vi "Encode PID Parameters.vi"(8 "ADD Parameters (in)":string, 9 "Scanner Settings In":T2={"Scan1"=1, "Scan2"=1, "Scan3"=1, "Scan4"=1, "Scan5"=1, "Scan6"=1, "Scan7"=1, "Scan8"=1, "Scan9"=1, "Scan10"=1, "Scan11"=1, "Scan12"=1, "Scan13"=1, "Scan14"=1, "Scan15"=1, "Scan16"=1} {"Scan16" scale=0.0..2.0; "Scan15" scale=0.0..2.0; "Scan14" scale=0.0..2.0; "Scan13" scale=0.0..2.0; "Scan12" scale=0.0..2.0; "Scan11" scale=0.0..2.0; "Scan10" scale=0.0..2.0; "Scan9" scale=0.0..2.0; "Scan8" scale=0.0..2.0; "Scan7" scale=0.0..2.0; "Scan6" scale=0.0..2.0; "Scan5" scale=0.0..2.0; "Scan4" scale=0.0..2.0; "Scan3" min=0 max=2 scale=0.0..2.0; "Scan2" min=0 max=2 scale=0.0..2.0; "Scan1" min=0 max=2 scale=0.0..2.0}, 10 "Internal Scanner Exists?":bool, 11 "PID Test Parameters In":T1={"Voltage (-2000~2000V)"=-1500, "High Limit(-20000~20000uA)"=0.0, "Low Limit(-20000~20000uA)"=0.0, "Ramp Up Time (0.1~999.9seconds)"=0.1, "Dwell Time (0, 0.4~999.9s, 0.1~999.9m/h)"=1.0, "Dwell Unit"=enum."second", "Ramp Down Time (0,1~999.9seconds)"=0.0} {"Ramp Down Time (0,1~999.9seconds)" format="%.1f"; "Dwell Time (0, 0.4~999.9s, 0.1~999.9m/h)" format="%.1f"; "Ramp Up Time (0.1~999.9seconds)" format="%.1f"; "Low Limit(-20000~20000uA)" format="%.1f"; "High Limit(-20000~20000uA)" format="%.1f"}) -> (1 "Scanner Settings Out":T2={"Scan1"=1, "Scan2"=1, "Scan3"=1, "Scan4"=1, "Scan5"=1, "Scan6"=1, "Scan7"=1, "Scan8"=1, "Scan9"=1, "Scan10"=1, "Scan11"=1, "Scan12"=1, "Scan13"=1, "Scan14"=1, "Scan15"=1, "Scan16"=1} {"Scan16" scale=0.0..2.0; "Scan15" scale=0.0..2.0; "Scan14" scale=0.0..2.0; "Scan13" scale=0.0..2.0; "Scan12" scale=0.0..2.0; "Scan11" scale=0.0..2.0; "Scan10" scale=0.0..2.0; "Scan9" scale=0.0..2.0; "Scan8" scale=0.0..2.0; "Scan7" scale=0.0..2.0; "Scan6" scale=0.0..2.0; "Scan5" scale=0.0..2.0; "Scan4" scale=0.0..2.0; "Scan3" min=0 max=2 scale=0.0..2.0; "Scan2" min=0 max=2 scale=0.0..2.0; "Scan1" min=0 max=2 scale=0.0..2.0}, 2 "PID Test Parameters Out":T1={"Voltage (-2000~2000V)"=-1500, "High Limit(-20000~20000uA)"=0.0, "Low Limit(-20000~20000uA)"=0.0, "Ramp Up Time (0.1~999.9seconds)"=0.1, "Dwell Time (0, 0.4~999.9s, 0.1~999.9m/h)"=1.0, "Dwell Unit"=enum."second", "Ramp Down Time (0,1~999.9seconds)"=0.1} {"Ramp Down Time (0,1~999.9seconds)" format="%.1f"; "Dwell Time (0, 0.4~999.9s, 0.1~999.9m/h)" format="%.1f"; "Ramp Up Time (0.1~999.9seconds)" format="%.1f"; "Low Limit(-20000~20000uA)" format="%.1f"; "High Limit(-20000~20000uA)" format="%.1f"}, 3 "ADD command":string)   [LabVIEW 2014, in "eec EST 300.lvlib"]
uses:
  <instrlib>/eec EST 300/eec EST 300.lvlib
  <instrlib>/eec EST 300/Public/Configure/Steps/Low Level/Scanner Settings.ctl
  <instrlib>/eec EST 300/Public/Configure/Steps/Low Level/PID Test Parameters.ctl
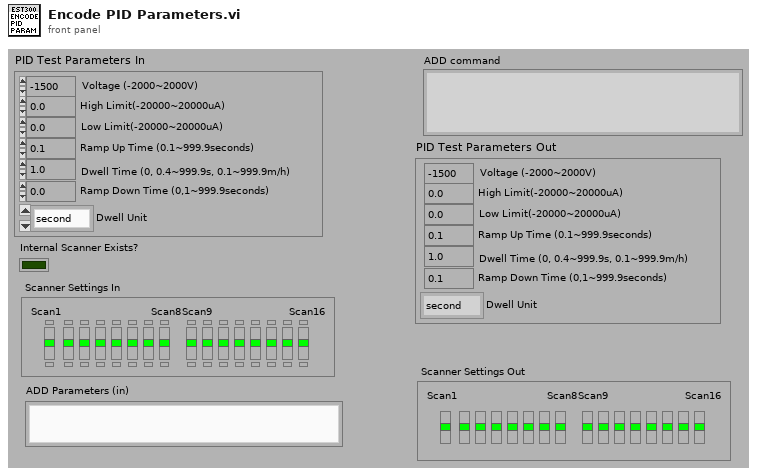
[diagram p1: front panel]
types:
  T1 = typedef "eec EST 300.lvlib/PID Test Parameters.ctl" = cluster{"Voltage (-2000~2000V)":i32, "High Limit(-20000~20000uA)":dbl, "Low Limit(-20000~20000uA)":dbl, "Ramp Up Time (0.1~999.9seconds)":dbl, "Dwell Time (0, 0.4~999.9s, 0.1~999.9m/h)":dbl, "Dwell Unit":enum16{"second", "minute", "hour"}, "Ramp Down Time (0,1~999.9seconds)":dbl}
  T2 = typedef "eec EST 300.lvlib/Scanner Settings.ctl" = cluster{"Scan1":i32, "Scan2":i32, "Scan3":i32, "Scan4":i32, "Scan5":i32, "Scan6":i32, "Scan7":i32, "Scan8":i32, "Scan9":i32, "Scan10":i32, "Scan11":i32, "Scan12":i32, "Scan13":i32, "Scan14":i32, "Scan15":i32, "Scan16":i32}
  T3 = typedef "EEC EST 300.lvlib/Scanner Settings.ctl" = cluster{"Scan1":i32, "Scan2":i32, "Scan3":i32, "Scan4":i32, "Scan5":i32, "Scan6":i32, "Scan7":i32, "Scan8":i32, "Scan9":i32, "Scan10":i32, "Scan11":i32, "Scan12":i32, "Scan13":i32, "Scan14":i32, "Scan15":i32, "Scan16":i32}
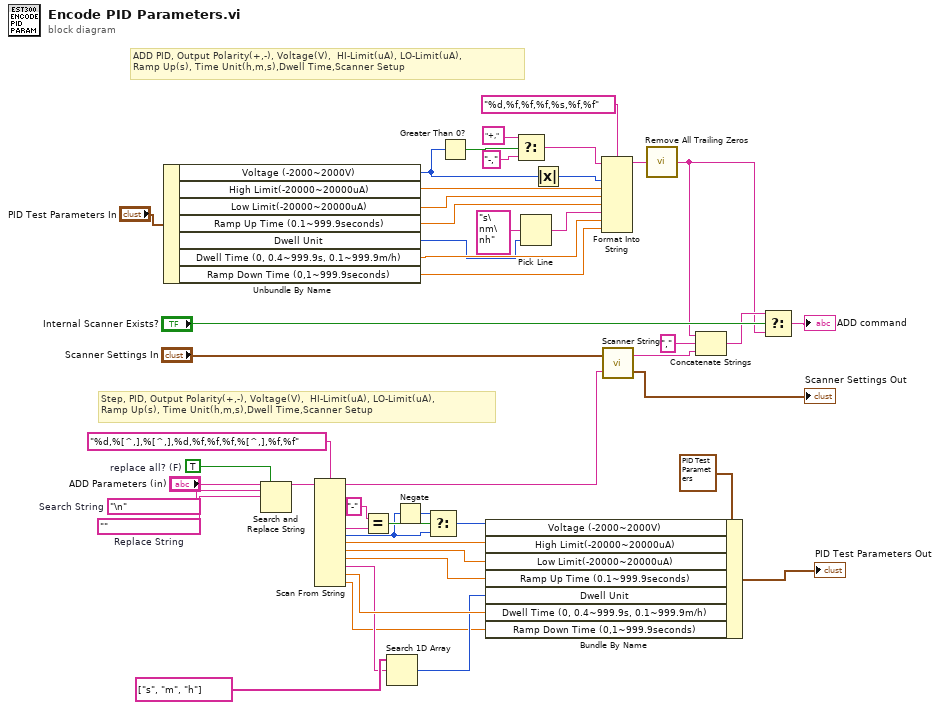
[diagram p0: block diagram]
diagram:
  w37 = TRUE  # replace all? (F)
  w38 = ""  # Replace String
  w39 = "\n"  # Search String
  # "Step, PID, Output Polarity(+,-), Voltage(V),  HI-Limit(uA), LO-Limit(uA), \nRamp Up(s), Time Unit(h,m,s),Dwell Time,Scanner Setup"
  # "ADD PID, Output Polarity(+,-), Voltage(V),  HI-Limit(uA), LO-Limit(uA), \nRamp Up(s), Time Unit(h,m,s),Dwell Time,Scanner Setup"
  n1 = Unbundle By Name("PID Test Parameters In") -> ("Voltage (-2000~2000V)"=w28:i32, "High Limit(-20000~20000uA)"=w48:dbl, "Low Limit(-20000~20000uA)"=w47:dbl, "Ramp Up Time (0.1~999.9seconds)"=w46:dbl, "Dwell Unit"=w6:enum16{"second", "minute", "hour"}, "Dwell Time (0, 0.4~999.9s, 0.1~999.9m/h)"=w45:dbl, "Ramp Down Time (0,1~999.9seconds)"=w1:dbl)
  n2 = Search and Replace String(replace all?=w37, input string="ADD Parameters (in)", search string=w39, replace string=w38) -> (result string=w35:string)  [unwired: 4 in, 3 out]
  n3 = Scan From String(format string="%d,%[^,],%[^,],%d,%f,%f,%f,%[^,],%f,%f" ("Format String"), input string=w35) -> (remaining string=w30:string, output 3=w21:string, output 4=w18:i32, output 5=w15:dbl, output 6=w14:dbl, output 7=w13:dbl, output 8=w4:string, output 9=w12:dbl, output 10=w2:dbl)  [unwired: 14 in, 2 out]
  n4 = Equal?(x="-", y=w21) -> (x = y?=w19:bool)
  n5 = Search 1D Array(1D array=string[] ["s", "m", "h"], element=w4) -> (index of element=w3:i32)  [unwired: 1 in]
  n6 = Negate(x=w18) -> (-x=w17:i32)
  n7 = Select(t=w17, s=w19, f=w18) -> (s? t:f=w16:i32)
  n8 = Greater Than 0?(x=w28) -> (x > 0?=w23:bool)
  n9 = Bundle By Name(cluster=T1 {"Voltage (-2000~2000V)"=-1500, "High Limit(-20000~20000uA)"=0.0, "Low Limit(-20000~20000uA)"=0.0, "Ramp Up Time (0.1~999.9seconds)"=0.1, "Dwell Time (0, 0.4~999.9s, 0.1~999.9m/h)"=1.0, "Dwell Unit"=enum."second", "Ramp Down Time (0,1~999.9seconds)"=0.1} ("PID Test Parameters Out"), "Voltage (-2000~2000V)"=w16, "High Limit(-20000~20000uA)"=w15, "Low Limit(-20000~20000uA)"=w14, "Ramp Up Time (0.1~999.9seconds)"=w13, "Dwell Unit"=w3, "Dwell Time (0, 0.4~999.9s, 0.1~999.9m/h)"=w12, "Ramp Down Time (0,1~999.9seconds)"=w2) -> (→"PID Test Parameters Out":T1)
  n10 = Select(t="+,", s=w23, f="-,") -> (s? t:f=w25:string)
  n11 = Pick Line(multi-line string="s\nm\nh" ("Time Unit"), line index=w6) -> (output string=w7:string)  [unwired: 1 in]
  n12 = Absolute Value(x=w28) -> (abs(x)=w27:i32)
  n13 = Format Into String(format string="%d,%f,%f,%f,%s,%f,%f" ("Format String"), initial string=w25, w27, w48, w47, w46, w7, w45, w1) -> (resulting string=w10:string)  [unwired: 1 in, 1 out]
  n14 = call <instrlib>:"Scanner String.vi"("Scanner String (in)"=w30, "Scanner Settings in"="Scanner Settings In") -> ("Scanner Settings out"=→"Scanner Settings Out":T3, "Scanner String (out)"=w33:string)
  n15 = call <instrlib>:"Remove All Trailing Zeros.vi"("String in"=w10) -> ("String out"=w9:string)
  n16 = Concatenate Strings(w9, "," ("Substring"), w33) -> (w41:string)
  n17 = Select(t=w41, s="Internal Scanner Exists?", f=w9) -> (s? t:f=→"ADD command":string)
